vi "MW gated average intensity.vi"(10 "Time":dbl, 11 "rate":dbl=100.0 format="%0.2f") -> (3 "Contrast (%)":dbl)   [LabVIEW 2012]
uses:
  <vilib>/DAQmx/read.llb/DAQmx Read (Counter 1D DBL 1Chan NSamp).vi
  <vilib>/DAQmx/create/channels.llb/DAQmx Create Channel (CI-Count Edges).vi
  <vilib>/DAQmx/configure/timing.llb/DAQmx Timing (Sample Clock).vi
  <vilib>/DAQmx/miscellaneous.llb/DAQmx Fill In Error Info.vi
  <resource>/objmgr/daqmx.rc
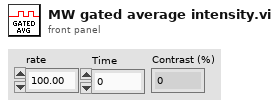
[diagram p1: front panel]
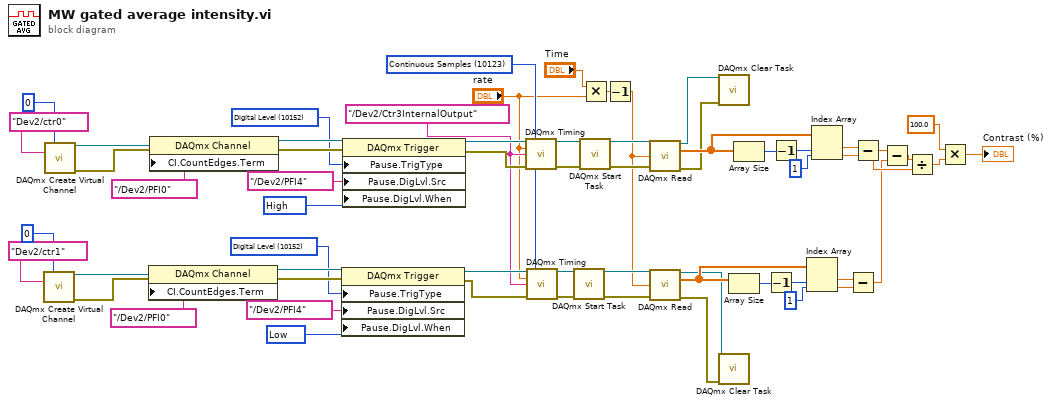
[diagram p0: block diagram]
diagram:
  w38 = tag "/Dev2/Ctr3InternalOutput" ("source")
  w37 = 10123 items=["Finite Samples"=10178, "Continuous Samples"=10123, "Hardware Timed Single Point"=12522] ("sample mode")
  w43 = 10214 items=["High"=10192, "Low"=10214] ("Pause.DigLvl.When")
  w45 = 10152 items=["Analog Level"=10101, "Analog Window"=10103, "Digital Level"=10152, "Digital Pattern"=10398, "None"=10230] ("Pause.TrigType")
  w52 = 10192 items=["High"=10192, "Low"=10214] ("Pause.DigLvl.When")
  w54 = 10152 items=["Analog Level"=10101, "Analog Window"=10103, "Digital Level"=10152, "Digital Pattern"=10398, "None"=10230] ("Pause.TrigType")
  n1 = call-poly <vilib>:"DAQmx Create Virtual Channel.vi"("initial count"=u32 0, "counter"=tag "Dev2/ctr1") -> ("task out"=w50:refnum<k21>, "error out"=w49:errorcluster)  [unwired: 12 in]
  n2 = call-poly <vilib>:"DAQmx Create Virtual Channel.vi"("initial count"=u32 0, "counter"=tag "Dev2/ctr0") -> ("task out"=w59:refnum<k21>, "error out"=w58:errorcluster)  [unwired: 12 in]
  n3 = property class="DAQmx Channel"(reference=w50, error in=w49, "CI.CountEdges.Term"=tag "/Dev2/PFI0") -> (reference out=w47:refnum<k21>, error out=w46:errorcluster)
  n4 = property class="DAQmx Channel"(reference=w59, error in=w58, "CI.CountEdges.Term"=tag "/Dev2/PFI0") -> (reference out=w56:refnum<k21>, error out=w55:errorcluster)
  n5 = property class="DAQmx Trigger"(reference=w47, error in=w46, "Pause.TrigType"=w45, "Pause.DigLvl.Src"=tag "/Dev2/PFI4", "Pause.DigLvl.When"=w43) -> (reference out=w40:refnum<k21>, error out=w39:errorcluster)
  n6 = property class="DAQmx Trigger"(reference=w56, error in=w55, "Pause.TrigType"=w54, "Pause.DigLvl.Src"=tag "/Dev2/PFI4", "Pause.DigLvl.When"=w52) -> (reference out=w42:refnum<k21>, error out=w41:errorcluster)
  n7 = call-poly <vilib>:"DAQmx Timing.vi"("task/channels in"=w42, "sample mode"=w37, "rate"="rate", "source"=w38, "error in"=w41) -> ("task out"=w36:refnum<k21>, "error out"=w13:errorcluster)  [unwired: 9 in]
  n8 = call-poly <vilib>:"DAQmx Timing.vi"("task/channels in"=w40, "sample mode"=w37, "rate"="rate", "source"=w38, "error in"=w39) -> ("task out"=w35:refnum<k21>, "error out"=w10:errorcluster)  [unwired: 9 in]
  n9 = call <vilib>:"DAQmx Start Task.vi"("task/channels in"=w35, "error in"=w10) -> ("task out"=w11:refnum<k21>, "error out"=w9:errorcluster)  [unwired: 12 in]
  n10 = call <vilib>:"DAQmx Start Task.vi"("task/channels in"=w36, "error in"=w13) -> ("task out"=w14:refnum<k21>, "error out"=w12:errorcluster)  [unwired: 12 in]
  n11 = Multiply(x="Time", y="rate") -> (x*y=w8:dbl)
  n12 = Decrement(x=w8) -> (x-1=w7:dbl)
  n13 = call-poly <vilib>:"DAQmx Read.vi"("task/channels in"=w14, "number of samples per channel"=w7, "error in"=w12) -> ("task out"=w6:refnum<k21>, "data"=w25:dbl[], "error out"=w5:errorcluster)  [unwired: 10 in]
  n14 = call-poly <vilib>:"DAQmx Read.vi"("task/channels in"=w11, "number of samples per channel"=w7, "error in"=w9) -> ("task out"=w4:refnum<k21>, "data"=w21:dbl[], "error out"=w3:errorcluster)  [unwired: 10 in]
  n15 = call <vilib>:"DAQmx Clear Task.vi"("task in"=w6, "error in"=w5) -> ()  [unwired: 13 in, 1 out]
  n16 = call <vilib>:"DAQmx Clear Task.vi"("task in"=w4, "error in"=w3) -> ()  [unwired: 13 in, 1 out]
  n17 = Array Size(array=w21) -> (size(s)=w30:i32)
  n18 = Array Size(array=w25) -> (size(s)=w32:i32)
  n19 = Decrement(x=w30) -> (x-1=w20:i32)
  n20 = Decrement(x=w32) -> (x-1=w27:i32)
  n21 = Index Array(array=w21, index #1=w20, index #2=1 ("index")) -> (element #1=w18:dbl, element #2=w29:dbl)
  n22 = Index Array(array=w25, index #1=w27, index #2=1 ("index")) -> (element #1=w24:dbl, element #2=w31:dbl)
  n23 = Subtract(x=w18, y=w29) -> (x-y=w17:dbl)
  n24 = Subtract(x=w24, y=w31) -> (x-y=w28:dbl)
  n25 = Subtract(x=w28, y=w17) -> (x-y=w16:dbl)
  n26 = Divide(x=w16, y=w28) -> (x/y=w23:dbl)
  n27 = Multiply(x=100.0, y=w23) -> (x*y=→"Contrast (%)":dbl)
